vi "DSDLL Initiate Digitizing Process.vi"(8 "error in":errorcluster, 11 "dsdll session in":T1) -> (0 "error out":errorcluster, 3 "dsdll session out":T1)   [LabVIEW 2018, in "DSDLL Virtual Digitizer.lvlib"]
doc: "Initiates acquisition. It creates data queue and starts digitizing process which runs on background. If succeds the process immediatelly starts digitizing and filling the queue with data. So this VI must be immediatelly followed by fetch loop that takes out data from the queue!"
uses:
  DSDLL Virtual Digitizer.lvlib
  DSDLL Session.ctl
  dsdll source distribution/dsdll_instance.ctl
  dsdll source distribution/dsdll_device_record.ctl
  DSDLL Process Config.ctl
  DSDLL Data Packet.ctl
  dsdll source distribution/dsdll.lvlib
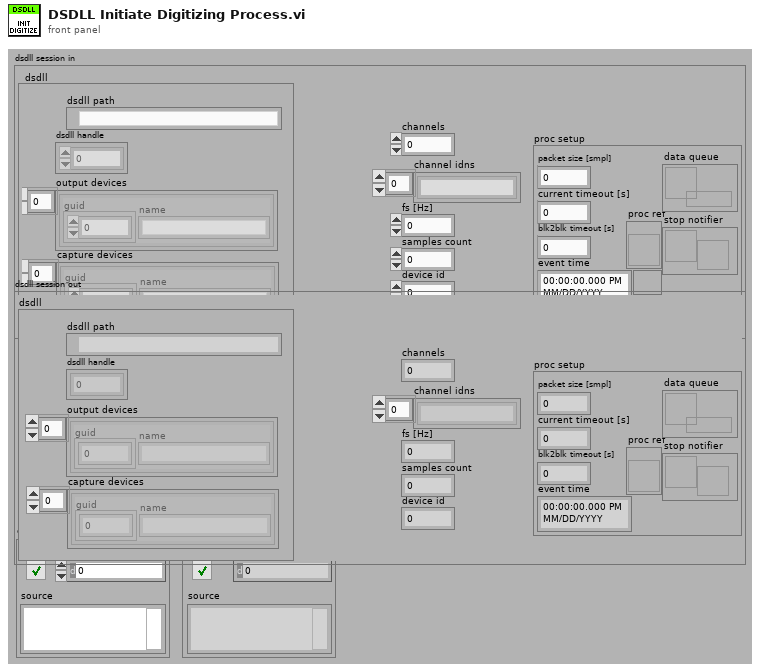
[diagram p1: front panel]
types:
  T1 = typedef "DSDLL Virtual Digitizer.lvlib/DSDLL Session.ctl" = cluster{"dsdll":T2, "channels":i32, "device id":i32, "channel idns":string[], "proc setup":T4, "samples count":i32, "fs [Hz]":dbl}
  T2 = typedef "dsdll.lvlib/dsdll_instance.ctl" = cluster{"dsdll path":path, "dsdll handle":u8[], "output devices":T3[], "capture devices":T3[]}
  T3 = typedef "dsdll.lvlib/dsdll_device_record.ctl" = cluster{"guid":u8[], "name":string}
  T4 = typedef "DSDLL Virtual Digitizer.lvlib/DSDLL Process Config.ctl" = cluster{"packet size [smpl]":i32, "current timeout [s]":dbl, "blk2blk timeout [s]":dbl, "event time":timestamp, "data queue":refnum<queue>, "stop notifier":refnum<notifier>, "proc ref":refnum<vi>}
  T5 = typedef "DSDLL Virtual Digitizer.lvlib/DSDLL Data Packet.ctl" = cluster{"int32":i32[][], "card buffer [%]":dbl, "all done?":bool, "offset [smpl]":i32, "sampling?":bool, "queue buffer [%]":dbl, "count [smpl]":i32, "valid?":bool}
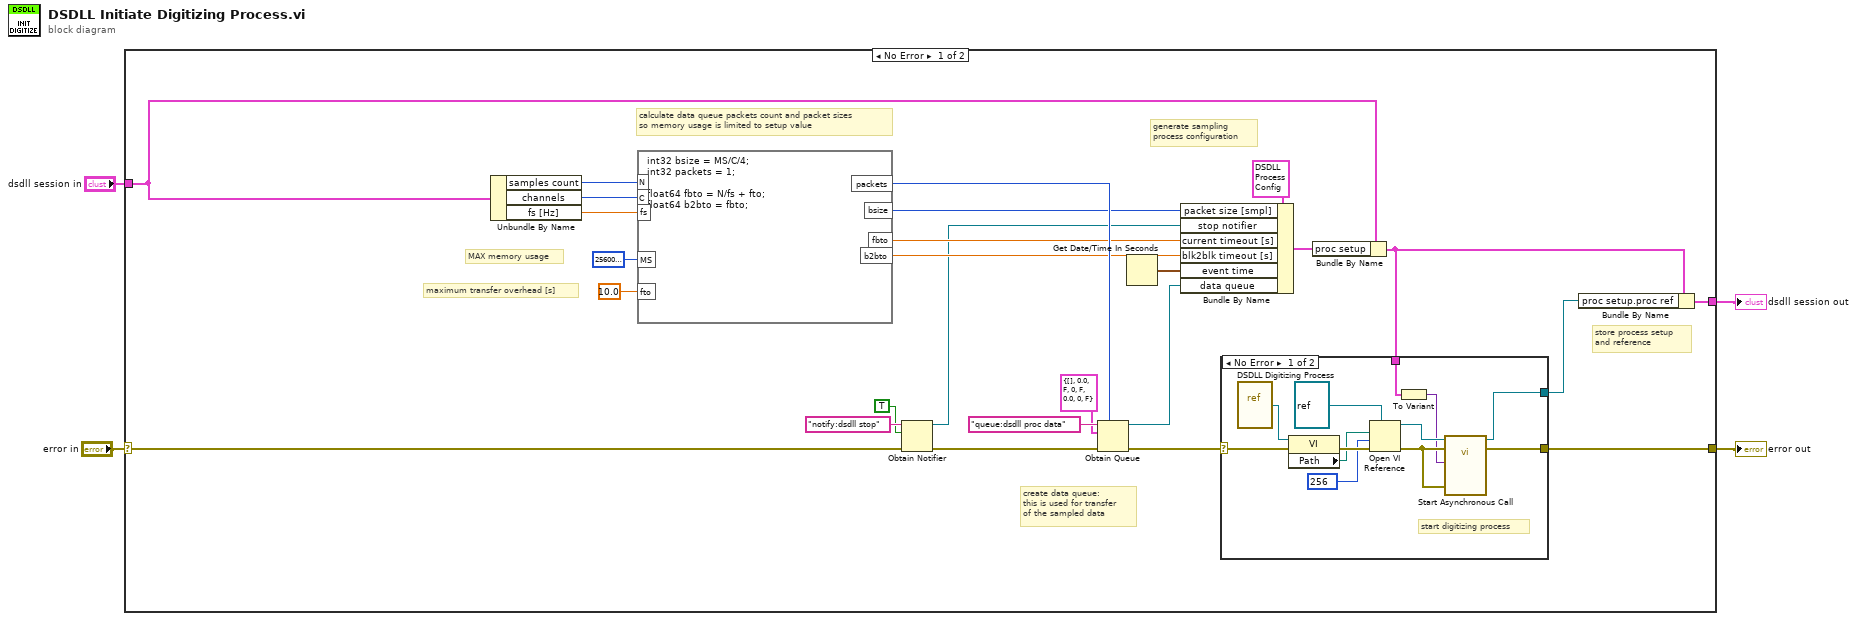
[diagram p0: block diagram]
diagram:
  n1 = case shown="No Error" "error in" {
    selector: "error in" -> [w7 w45]
    tunnel: [w9 w45] -> w4
    tunnel: "dsdll session in" -> [w12 w44]
    tunnel: [w18 w44] -> w2
    frame No Error {
      # "store process setup\nand reference"
      # "maximum transfer overhead [s]"
      # "generate sampling\nprocess configuration"
      # "calculate data queue packets count and packet sizes\nso memory usage is limited to setup value"
      # "MAX memory usage"
      # "create data queue:\nthis is used for transfer\nof the sampled data"
      n2 = Unbundle By Name(w12) -> ("samples count"=w28:i32, "channels"=w27:i32, "fs [Hz]"=w6:dbl)
      n3 = formula code="int32 bsize = MS/C/4;\nint32 packets = 1;\n\nfloat64 fbto = N/fs + fto;\nfloat64 b2bto = fbto;"("N"=w28, "C"=w27, "MS"=256000000 ("y"), "fto"=10.0 ("input variable"), "fs"=w6) -> ("packets"=w25:i32, "bsize"=w24:i32, "fbto"=w21:dbl, "b2bto"=w19:dbl)
      n4 = Obtain Notifier(name (unnamed)="notify:dsdll stop", notification data type=TRUE, error in (no error)=w7) -> (notifier out=w13:refnum<notifier>, error out=w15:errorcluster)  [unwired: 1 in, 1 out]
      n5 = Obtain Queue(max queue size (-1, unlimited)=w25, name (unnamed)="queue:dsdll proc data", element data type=T5 {"int32"=[], "card buffer [%]"=0.0, "all done?"=FALSE, "offset [smpl]"=0, "sampling?"=FALSE, "queue buffer [%]"=0.0, "count [smpl]"=0, "valid?"=FALSE} ("niScope packet"), error in (no error)=w15) -> (queue out=w5:refnum<queue>, error out=w23:errorcluster)  [unwired: 1 in, 1 out]
      n6 = Get Date/Time In Seconds() -> (seconds since 1Jan1904=w20:timestamp)
      n7 = Bundle By Name(cluster=T4 {"packet size [smpl]"=0, "current timeout [s]"=0.0, "blk2blk timeout [s]"=0.0, "event time"=timestamp(0 s since 1904-01-01), "data queue"=refnum, "stop notifier"=refnum, "proc ref"=refnum} ("setup"), "packet size [smpl]"=w24, "stop notifier"=w13, "current timeout [s]"=w21, "blk2blk timeout [s]"=w19, "event time"=w20, "data queue"=w5) -> (w11:T4)
      n8 = Bundle By Name(cluster=w12, "proc setup"=w11) -> (w8:T1)
      n9 = case shown="No Error" w23 {
        selector: w23 -> [w33 w43]
        tunnel: [w34 w43] -> w9
        tunnel: [w32 _] -> w10
        tunnel: w8 -> [w31 _]
        frame No Error {
          # "start digitizing process"
          n10 = vi-ref "DSDLL Digitizing Process.vi"() -> (w41:refnum<vi>)
          n11 = property class="VI"(reference=w41, error in=w33) -> (error out=w40:errorcluster, "Path"=w38:path)  [unwired: 1 out]
          n12 = Open VI Reference(type specifier VI Refnum (for type only)=refnum<vi> refnum, vi path=w38, options=256, error in (no error)=w40) -> (vi reference=w42:refnum<vi>, error out=w39:errorcluster)  [unwired: 2 in]
          n13 = To Variant(anything=w31) -> (Variant=w35:variant)
          n14 = call-by-ref "Start Asynchronous Call"(reference=w42, error in=w39, "error in"=w39, "niScope session"=w35) -> (reference out=w32:refnum<vi>, error out=w34:errorcluster)  [unwired: 8 in, 2 out]
        }
        frame Error {
        }
      }
      n15 = Bundle By Name(cluster=w8, "proc setup.proc ref"=w10) -> (w18:T1)
    }
    frame Error {
    }
  }
  "error out" <- w4
  "dsdll session out" <- w2
